vi "Configure Range Table (Spurious Emissions - IF Gain).vi"(0 "VISA resource name":refnum<visa-resource-name>, 1 "Auto IF Gain List":bool[](array[boolean])=[FALSE, FALSE], 5 "Manual IF Gain List":i32[](array[ring])=[0, 0] items=["Low Gain", "High Gain"], 11 "error in (no error)":errorcluster) -> (4 "VISA resource name out":refnum<visa-resource-name>, 15 "error out":errorcluster)   [LabVIEW 2018, in "Agilent MXA Series.lvlib"]
doc: "Configures the IF Gain settings under Range Table for Spurious Emissions measurement type."
uses:
  Agilent MXA Series.lvlib
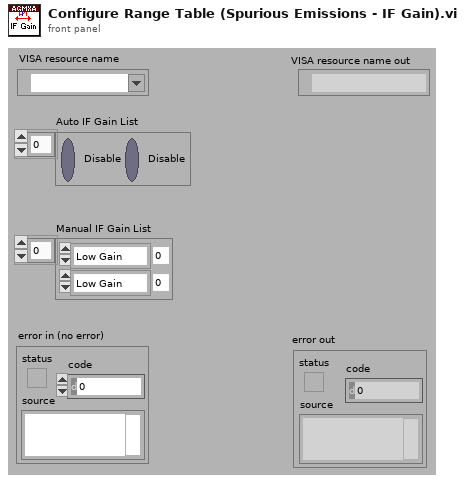
[diagram p1: front panel]
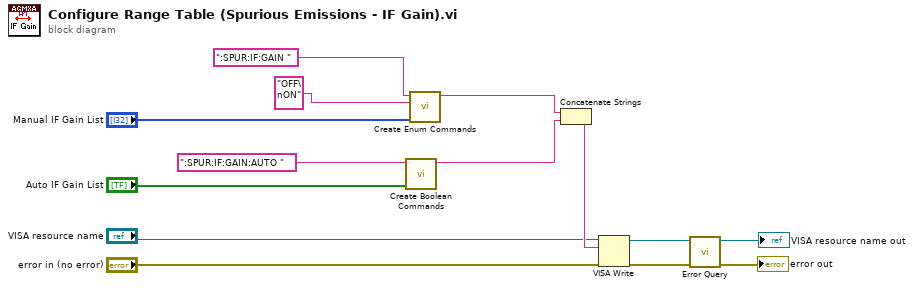
[diagram p0: block diagram]
diagram:
  n1 = call "Create Boolean Commands.vi"("Boolean States"="Auto IF Gain List", "Command"=":SPUR:IF:GAIN:AUTO ") -> ("Result String"=w5:string)  [unwired: 9 in]
  n2 = call "Create Enum Commands.vi"("Enum Values"="Manual IF Gain List", "Multi-line Text"="OFF\nON" ("multi-line string"), "Commands"=":SPUR:IF:GAIN ") -> ("Result"=w1:string)  [unwired: 8 in]
  n3 = Concatenate Strings(w1, w5) -> (w12:string)
  n4 = VISA Write(VISA resource name="VISA resource name", write buffer=w12, error in (no error)="error in (no error)") -> (VISA resource name out=w11:refnum<visa-resource-name>, error out=w10:errorcluster)  [unwired: 1 out]
  n5 = call "Error Query.vi"("error in (no error)"=w10, "VISA resource name"=w11) -> ("error out"=→"error out":errorcluster, "VISA resource name out"=→"VISA resource name out":refnum<visa-resource-name>)  [unwired: 6 in, 2 out]
